vi "run_cmd_file.vi"(7 "configuration":T1={"username"="", "password"="", "host"="", "type"=enum."ssh"}, 8 "error in (no error)":errorcluster, 11 "shell_script":path) -> (0 "error out":errorcluster, 3 "standard_output":string)   [LabVIEW 2015, in "lv-bin-plink.lvlib" / "v1.lvlib"]
uses:
  v1.lvlib
  _controls/configuration.ctl
  _controls/type.ctl
  <userlib>/antonio-alexander/lv-bin/public/api/v1/v1.lvlib
  lv-bin-plink.lvlib
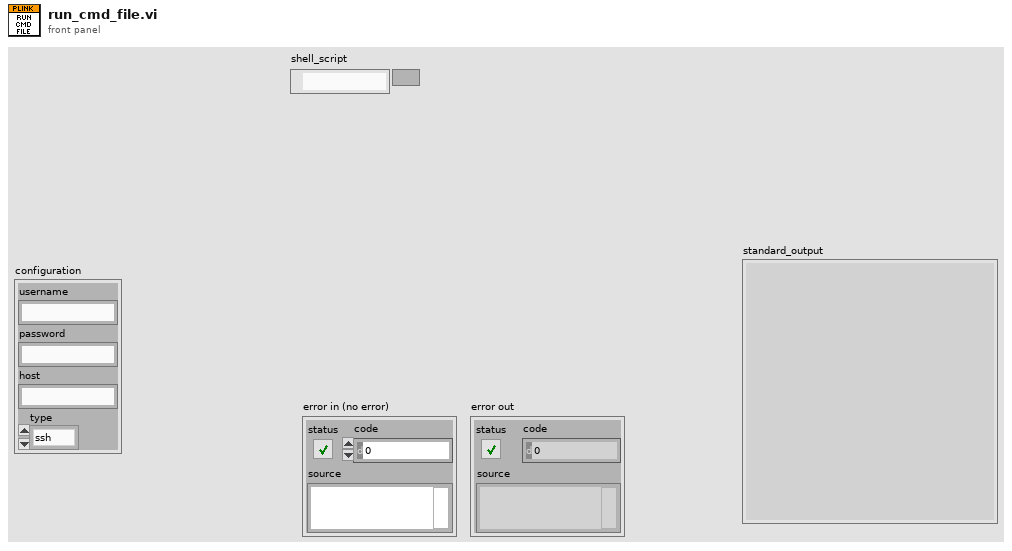
[diagram p1: front panel]
types:
  T1 = typedef "lv-bin-plink.lvlib/v1.lvlib/configuration.ctl" = cluster{"username":string, "password":string, "host":string, "type":T2}
  T2 = typedef "lv-bin-plink.lvlib/v1.lvlib/type.ctl" = enum16{"<type>", "ssh", "telnet", "rlogin", "raw", "serial"}
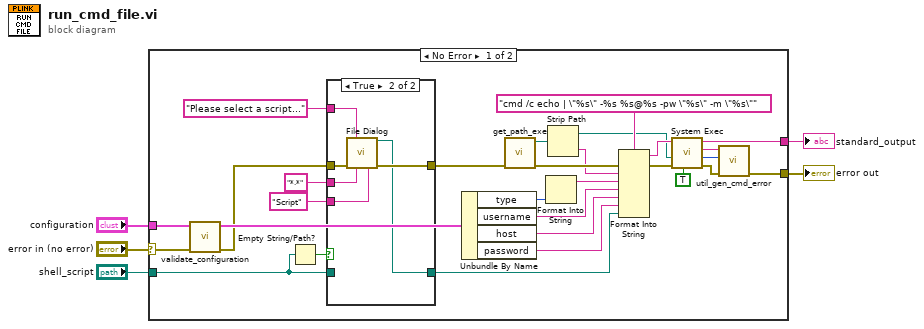
[diagram p0: block diagram]
diagram:
  n1 = case shown="No Error" "error in (no error)" {
    selector: "error in (no error)" -> [w8 w43]
    tunnel: "configuration" -> [w10 _]
    tunnel: [w34 w43] -> w4
    tunnel: [w33 _] -> w3
    tunnel: "shell_script" -> [w31 _]
    frame No Error {
      n2 = call "validate_configuration.vi"("error in (no error)"=w8, "configuration in"=w10) -> ("error out"=w7:errorcluster, "configuration out"=w9:T1)  [unwired: 8 in]
      n3 = Empty String/Path?(string/path=w31) -> (empty?=w32:bool)
      n4 = case shown="True" w32 {
        tunnel: [w35 w42] -> w12
        tunnel: w31 -> [w36 _]
        tunnel: "Please select a script..." ("prompt") -> [_ w41]
        tunnel: [w36 w40] -> w11
        tunnel: "*.*" ("pattern (all files)") -> [_ w39]
        tunnel: "Script" ("pattern label") -> [_ w38]
        tunnel: w7 -> [w35 w37]
        frame False {
        }
        frame True {
          n5 = call "File Dialog"("prompt"=w41, "error in"=w37, "pattern (all files)"=w39, "pattern label"=w38) -> ("selected path"=w40:path, "error out"=w42:errorcluster)  [unwired: 8 in, 2 out]
        }
      }
      n6 = Unbundle By Name(w9) -> ("type"=w20:T2, "username"=w18:string, "host"=w17:string, "password"=w16:string)
      n7 = call "get_path_exe.vi"("error in (no error)"=w12) -> ("error out"=w21:errorcluster, "plink"=w14:path)  [unwired: 9 in]
      n8 = Format Into String(w20) -> (resulting string=w19:string)  [unwired: 3 in, 1 out]
      n9 = Strip Path(path=w14) -> (stripped path=w15:path, name=w13:string)
      n10 = Format Into String(format string="cmd /c echo | \"%s\" -%s %s@%s -pw \"%s\" -m \"%s\"", error in=w21, w13, w19, w18, w17, w16, w11) -> (resulting string=w26:string, error out=w25:errorcluster)  [unwired: 1 in]
      n11 = call <vilib>:"System Exec.vi"("run minimized? (F)"=TRUE, "error in (no error)"=w25, "working directory"=w15, "command line"=w26) -> ("error out"=w23:errorcluster, "return code"=w6:i32, "standard error"=w24:string, "standard output"=w33:string)  [unwired: 4 in]
      n12 = call <userlib>:"util_gen_cmd_error.vi"("error in (no error)"=w23, "return_code"=w6, "standard_error"=w24) -> ("error out"=w34:errorcluster)  [unwired: 8 in]
    }
    frame Error {
    }
  }
  "error out" <- w4
  "standard_output" <- w3
